vi "xiC - IMAQ - Tree_MenuSelection.vi"(6 "SelectedMenuTag":string, 8 "error in (no error)":errorcluster, 11 "Attributes In":T1) -> (0 "error out":errorcluster, 3 "Attributes Out":T1)   [LabVIEW 2013]
uses:
  xiC - IMAQ - Attributes.ctl
  C:/Projects/Cameras3.x/xiLib/xiLIB_64bit/xiLIB/xiCamLib/API/x64/xiApi.NETX64.dll
  xiLIB_64bit/xiLIB/xiCamLib/API/x64/xiApi.NETX64.dll
  xiC - IMAQ - TreeDisplayType.ctl
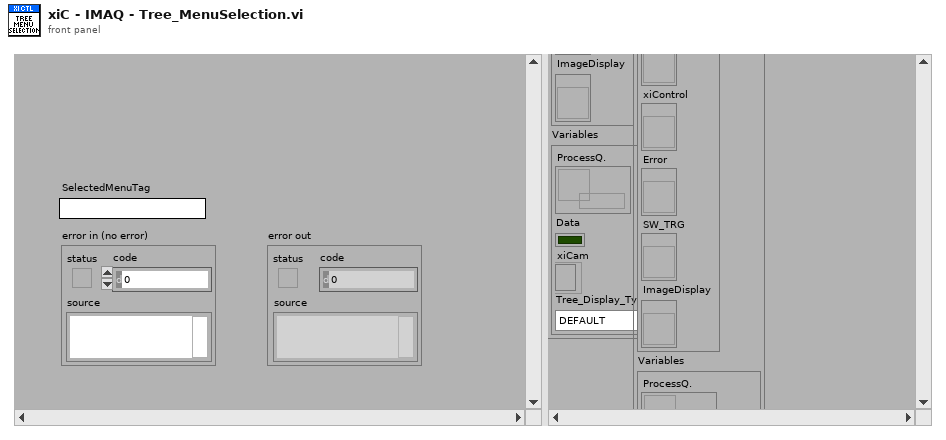
[diagram p1: front panel]
types:
  T1 = typedef "xiC - IMAQ - Attributes.ctl" = cluster{"Controls":cluster{"VI Ref.":refnum<vi>, "Tree":refnum<vi>, "Info":refnum<vi>, "PRMName":refnum<vi>, "xiControl":refnum<vi>, "Error":refnum<vi>, "SW_TRG":refnum<vi>, "ImageDisplay":refnum<vi>}, "Variables":cluster{"ProcessQ.":refnum<queue>, "Data":bool, "xiCam":refnum<k24>, "Tree_Display_Type":T2}}
  T2 = typedef "xiC - IMAQ - TreeDisplayType.ctl" = enum16{"DEFAULT", "HIDE_MAX_MIN"}
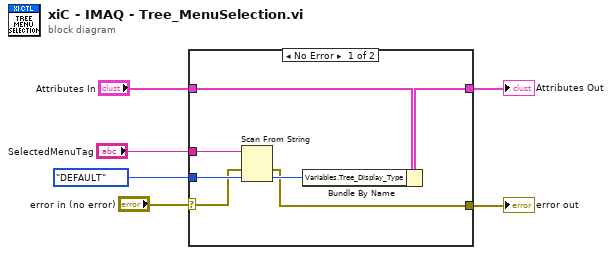
[diagram p0: block diagram]
diagram:
  n1 = case shown="No Error" "error in (no error)" {
    selector: "error in (no error)" -> [w8 w15]
    tunnel: [w7 w15] -> w5
    tunnel: "Attributes In" -> [w10 w14]
    tunnel: [w9 w14] -> w3
    tunnel: "SelectedMenuTag" -> [w13 _]
    tunnel: xiC_-_IMAQ_-_TreeDisplayType."DEFAULT" ("Symbol_Type") -> [w12 _]
    frame No Error {
      n2 = Scan From String(input string=w13, error in=w8, default 1=w12) -> (error out=w7:errorcluster, output 1=w11:T2)  [unwired: 2 in, 2 out]
      n3 = Bundle By Name(cluster=w10, "Variables.Tree_Display_Type"=w11) -> (w9:T1)
    }
    frame Error {
    }
  }
  "error out" <- w5
  "Attributes Out" <- w3
